vi "set_channel_index_on_device.vi"(8 "error in (no error)":errorcluster, 10 "channel index on device":i32, 11 "DAQmxWriteSignals.lvclass in":refnum<class "SignalWriterMM140725DAQmx.lvclass">) -> (0 "error out":errorcluster, 3 "DAQmxWriteSignals.lvclass out":refnum<class "SignalWriterMM140725DAQmx.lvclass">)   [LabVIEW 2010, in "SignalWriterMM140725DAQmx.lvclass"]
uses:
  SignalWriterMM140725DAQmx.lvclass
  SignalWriterMM140725DAQmx.lvclass/SignalWriterMM140725DAQmx.ctl
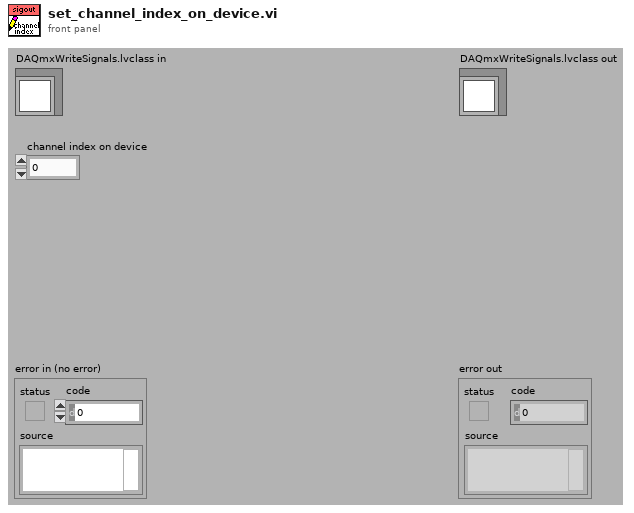
[diagram p1: front panel]
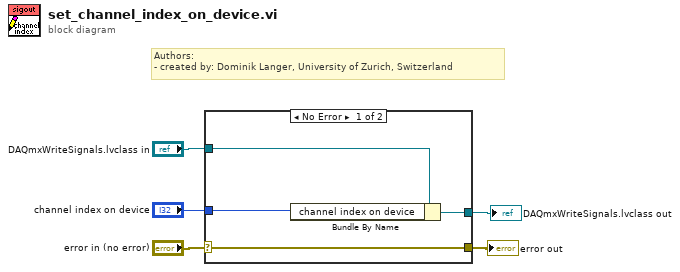
[diagram p0: block diagram]
diagram:
  # "Authors: \n- created by: Dominik Langer, University of Zurich, Switzerland"
  n1 = case shown="No Error" "error in (no error)" {
    selector: "error in (no error)" -> [w9 w10]
    tunnel: [w9 w10] -> w4
    tunnel: [w7 w11] -> w2
    tunnel: "DAQmxWriteSignals.lvclass in" -> [w8 w11]
    tunnel: "channel index on device" -> [w6 _]
    frame No Error {
      n2 = Bundle By Name(cluster=w8, "channel index on device"=w6) -> (w7:refnum<class "SignalWriterMM140725DAQmx.lvclass">)
    }
    frame Error {
    }
  }
  "error out" <- w4
  "DAQmxWriteSignals.lvclass out" <- w2
